vi "Tosca-Init Data Analysis.vi"(0 "Tosca":refnum<class "Parameters.lvclass">, 2 "IPC":T2, 9 "Control Refs":T1, 11 "error in (no error)":errorcluster, 12 "Session Info":T3={"Animal ID"="", "Session"=1, "Path"=path "", "Run"=0} {"Session" min=1 step=1}) -> (3 "Run":i32, 4 "Tosca out":refnum<class "Parameters.lvclass">, 13 "Session Info out":T3={"Animal ID"="", "Session"=1, "Path"=path "", "Run"=0} {"Session" min=1 step=1}, 14 "Analysis":T4, 15 "error out":errorcluster)   [LabVIEW 2020]
uses:
  Typedefs/Tosca-Session Info.ctl
  Typedefs/Tosca-Analysis State.ctl
  Typedefs/Tosca-Adaptation State.ctl
  Typedefs/Tosca-Adaptation Track State.ctl
  Typedefs/Tosca-Adaptation History Element.ctl
  Classes/Parameters/Histogram Data.ctl
  Classes/Parameters/Connect.ctl
  IPC VIs/Tosca-IPC.ctl
  Classes/Parameters/Parameters.lvclass
  Digital Input VIs/Tosca-DI Queue Data.ctl
  Digital Input VIs/Tosca-Input Event.ctl
  Digital Input VIs/Tosca-Input Criterion.ctl
  epl-vi-lib/Utility VIs/Type Defs/Logic State.ctl
  Typedefs/Tosca-Accumulator.ctl
  Typedefs/Tosca-State AODO.ctl
  Typedefs/Tosca-AO Runtime.ctl
  Typedefs/Tosca-DO Runtime.ctl
  epl-vi-lib/Signal Synthesis VIs/4th Generation/Classes/SignalManager/SignalManager.lvclass
  Typedefs/Tosca-Synapse Start Data.ctl
  IPC VIs/Tosca-Message.ctl
  IPC VIs/Tosca-Message Action.ctl
  Typedefs/Tosca-Thread Type.ctl
  Imaging VIs/Tosca-2P-Notifier Data.ctl
  Typedefs/Tosca-MATLAB Queue Data.ctl
  Visual Stim VIs/Tosca-Grating.ctl
  Visual Stim VIs/Tosca-Grating Type.ctl
  Typedefs/Tosca-File IO Notification.ctl
  Typedefs/Tosca-Control Refs.ctl
  FSM Graph VIs/LV Source/FSM Editor/FSM Editor.xctl
  Classes/Parameters/Parameters.lvclass/Parameters.ctl
  Classes/Parameters/Read MATLAB function.vi
  Classes/Parameters/Read Connect.vi
  Classes/Parameters/Read AI.vi
  Tosca-Globals.vi
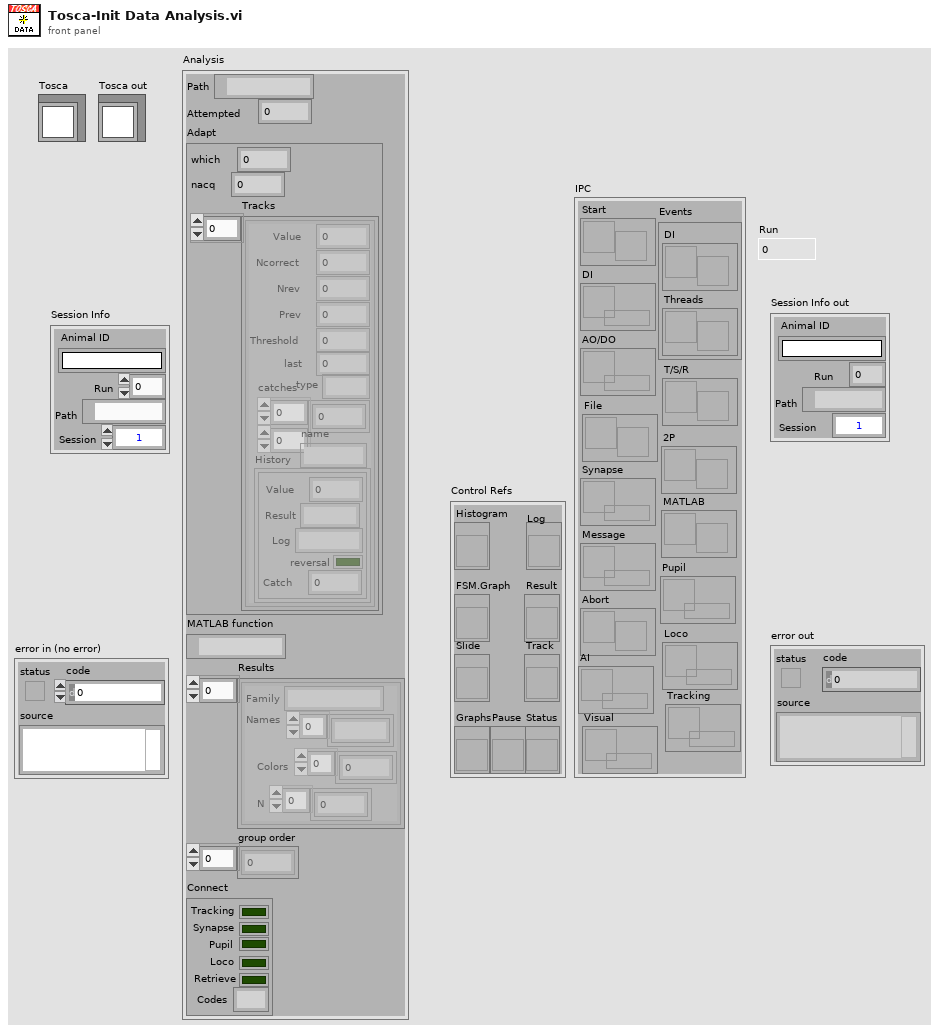
[diagram p1: front panel]
types:
  T1 = typedef "Tosca-Control Refs.ctl" = cluster{"FSM.Graph":refnum<vi>, "Slide":refnum<vi>, "Result":refnum<vi>, "Histogram":refnum<vi>, "Graphs":refnum<vi>, "Track":refnum<vi>, "Log":refnum<vi>, "Status":refnum<vi>, "Pause":refnum<vi>}
  T2 = typedef "Tosca-IPC.ctl" = cluster{"Start":refnum<notifier>, "DI":refnum<queue>, "AO/DO":refnum<queue>, "Synapse":refnum<queue>, "Message":refnum<queue>, "Abort":refnum<notifier>, "Events":cluster{"DI":refnum<user-event>, "Threads ":refnum<user-event>}, "T/S/R":refnum<notifier>, "2P":refnum<notifier>, "MATLAB":refnum<notifier>, "Pupil":refnum<queue>, "Loco":refnum<queue>, "AI":refnum<queue>, "Tracking":refnum<queue>, "Visual":refnum<queue>, "File":refnum<notifier>}
  T3 = typedef "Tosca-Session Info.ctl" = cluster{"Animal ID":string, "Session":i32, "Path":path, "Run":i32}
  T4 = typedef "Tosca-Analysis State.ctl" = cluster{"Path":path, "Attempted":i32, "Adapt":T5, "MATLAB function":path, "Results":T8[], "group order":i32[], "Connect":T9}
  T5 = typedef "Tosca-Adaptation State.ctl" = cluster{"which":i32, "nacq":i32, "Tracks":T6[]}
  T6 = typedef "Tosca-Adaptation Track State.ctl" = cluster{"Value":dbl, "Ncorrect":i32, "Nrev":i32, "Prev":dbl, "History":T7[], "Threshold":dbl, "last":i32, "type":string, "catches":dbl[][], "name":string}
  T7 = typedef "Tosca-Adaptation History Element.ctl" = cluster{"Value":dbl, "Result":string, "Log":string, "reversal":bool, "Catch":dbl}
  T8 = typedef "Parameters.lvclass/Histogram Data.ctl" = cluster{"Family":string, "Names":string[], "Colors":u32[], "N":i32[]}
  T9 = typedef "Parameters.lvclass/Connect.ctl" = cluster{"Tracking":bool, "Synapse":bool, "Pupil":bool, "Loco":bool, "Retrieve":bool, "Codes":string}
  T10 = typedef "Tosca-File IO Notification.ctl" = cluster{"Operation":enum16{"Start", "Update", "Finish"}, "Filestem":string}
  T11 = typedef "Tosca-AI.ctl" = cluster{"active":bool, "Fs":dbl, "AI":string[], "DI":string[]}
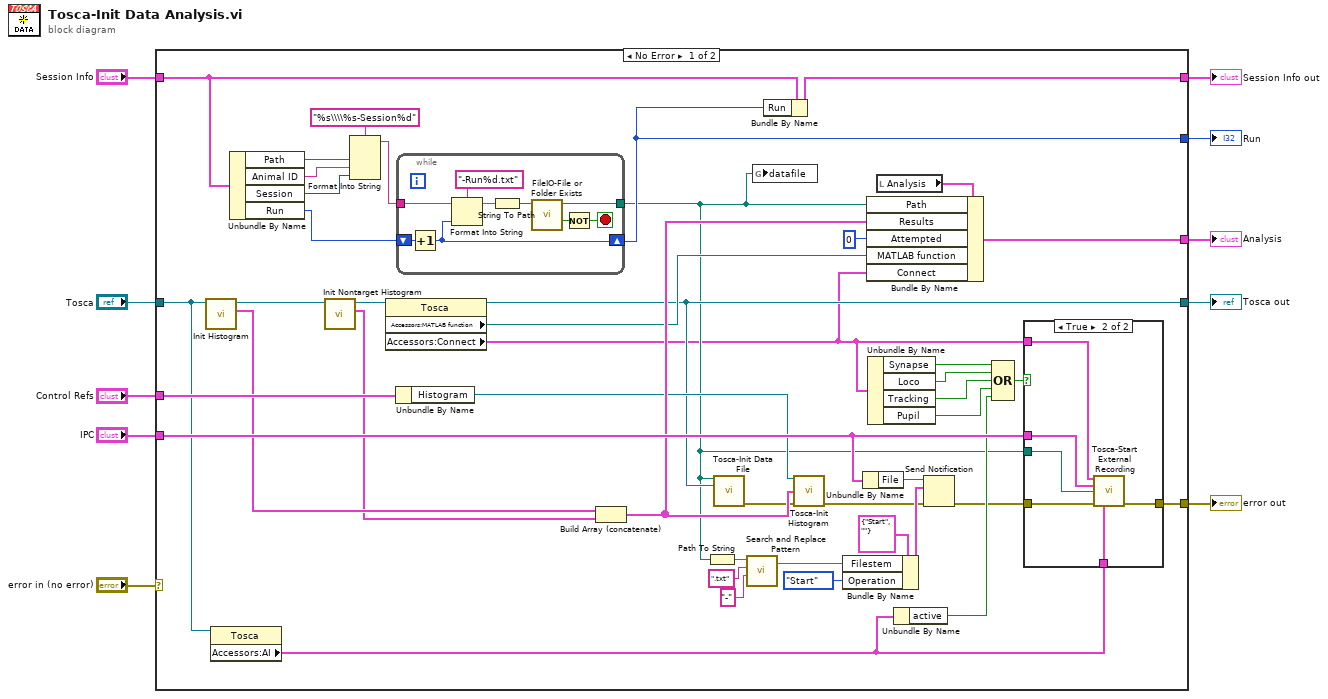
[diagram p0: block diagram]
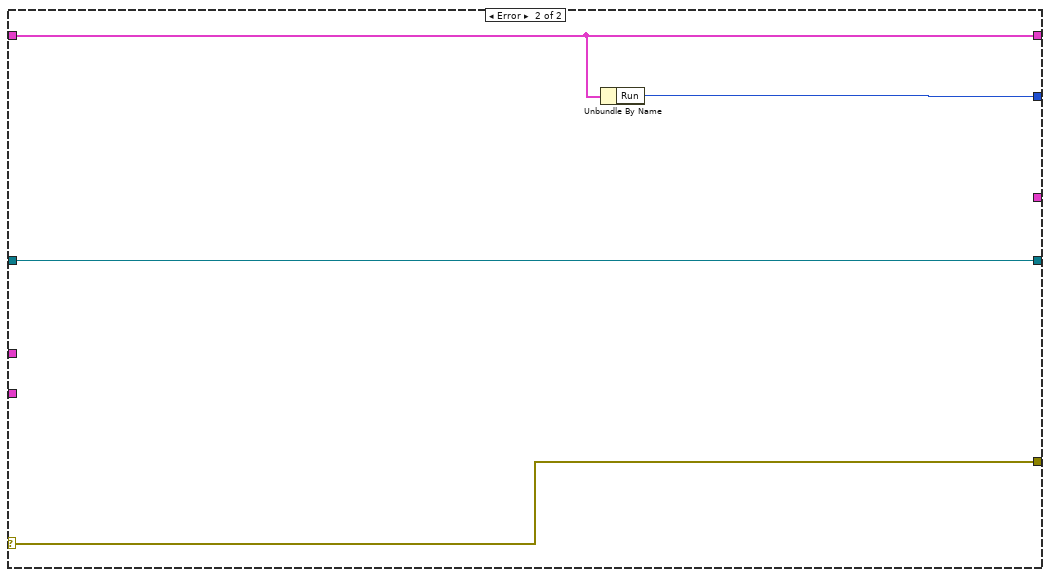
[diagram p3: hidden frame]
diagram:
  n1 = case shown="No Error" "error in (no error)" {
    selector: "error in (no error)" -> [_ w74]
    tunnel: [w34 w74] -> w9
    tunnel: "Session Info" -> [w45 w73]
    tunnel: [w47 _] -> w7
    tunnel: [w44 w73] -> w6
    tunnel: [w37 w72] -> w5
    tunnel: "IPC" -> [w33 _]
    tunnel: "Control Refs" -> [w30 _]
    tunnel: "Tosca" -> [w20 w71]
    tunnel: [w18 w71] -> w1
    frame No Error {
      n2 = call "Init Histogram.vi"("Tosca in"=w20) -> ("Data"=w19:T8[], "Tosca out"=w16:refnum<class "Parameters.lvclass">)  [unwired: 8 in, 1 out]
      n3 = property class="Tosca"(reference=w20) -> ("Accessors:AI"=w21:T11)  [unwired: 1 in, 2 out]
      n4 = Unbundle By Name(w45) -> ("Path"=w53:path, "Animal ID"=w52:string, "Session"=w51:i32, "Run"=w49:i32)
      n5 = call "Init Nontarget Histogram.vi"("Tosca in"=w16) -> ("Data"=w14:T8, "Tosca out"=w15:refnum<class "Parameters.lvclass">)  [unwired: 8 in, 1 out]
      n6 = Format Into String(format string="%s\\\\%s-Session%d", w53, w52, w51) -> (resulting string=w50:string)  [unwired: 2 in, 1 out]
      n7 = property class="Tosca"(reference=w15) -> (reference out=w18:refnum<class "Parameters.lvclass">, "Accessors:MATLAB function"=w23:path, "Accessors:Connect"=w13:T9)  [unwired: 1 in, 1 out]
      n8 = Unbundle By Name(w30) -> ("Histogram"=w29:refnum<vi>)
      n9 = while {
        tunnel: w50 -> [w68]
        tunnel: [w64] -> w17
        shift-right: [w66] -> w37
        shift-left: w49 -> [w67]
        stop <- w63 stop-if-true
        n10 = Increment(x=w67) -> (x+1=w66:i32)
        n11 = Format Into String(format string="-Run%d.txt", initial string=w68, w66) -> (resulting string=w69:string)  [unwired: 1 in, 1 out]
        n12 = String To Path(string=w69) -> (path=w65:path)
        n13 = call "FileIO-File or Folder Exists.vi"("path"=w65) -> ("Exists?"=w62:bool, "dup path"=w64:path)  [unwired: 7 in, 2 out]
        n14 = Not(x=w62) -> (.not. x?=w63:bool)
      }
      n15 = Build Array (concatenate)(w19, w14) -> (w31:T8[])
      n16 = Path To String(path=w17) -> (string=w38:string)
      n17 = call "Tosca-Init Data File.vi"("Path"=w17, "Tosca"=w18) -> ("error out"=w11:errorcluster)  [unwired: 13 in]
      n18 = call <vilib>:"Search and Replace Pattern.vi"("string"=w38, "regular expression (\"\")"=".txt" ("regular expression (\"\")"), "replace string (\"\")"="-" ("replace string (\"\")")) -> ("result string"=w36:string)  [unwired: 2 in, 1 out]
      n19 = global write "Tosca-Globals.vi" "datafile"(w17) -> ()
      n20 = Bundle By Name(cluster=w45, "Run"=w37) -> (w44:T3)
      n21 = call "Tosca-Init Histogram.vi"("Histogram"=w29, "Results"=w31, "error in (no error)"=w11) -> ("error out"=w32:errorcluster)  [unwired: 12 in]
      n22 = Bundle By Name(cluster=T10 {"Operation"=enum."Start", "Filestem"=""} ("element"), "Filestem"=w36, "Operation"=enum16{"Start", "Update", "Finish"}."Start") -> (w42:T10)
      n23 = Unbundle By Name(w33) -> ("File"=w35:refnum<notifier>)
      n24 = Unbundle By Name(w13) -> ("Synapse"=w28:bool, "Loco"=w27:bool, "Tracking"=w25:bool, "Pupil"=w22:bool)
      n25 = local read "Analysis"() -> (w48:T4)
      n26 = Bundle By Name(cluster=w48, "Path"=w17, "Results"=w31, "Attempted"=0, "MATLAB function"=w23, "Connect"=w13) -> (w47:T4)
      n27 = Unbundle By Name(w21) -> ("active"=w24:bool)
      n28 = Send Notification(notification=w42, notifier=w35, error in (no error)=w32) -> (error out=w12:errorcluster)  [unwired: 1 out]
      n29 = Compound Arithmetic op=OR(w28, w27, w25, w22, w24) -> (w26:bool)
      n30 = case shown="True" w26 {
        tunnel: w13 -> [_ w56]
        tunnel: w12 -> [w55 w61]
        tunnel: [w55 w60] -> w34
        tunnel: w33 -> [_ w59]
        tunnel: w17 -> [_ w58]
        tunnel: w21 -> [_ w57]
        frame False {
        }
        frame True {
          n31 = call "Tosca-Start External Recording.vi"("Connect"=w56, "IPC"=w59, "Path"=w58, "error in (no error)"=w61, "AI"=w57) -> ("error out"=w60:errorcluster)  [unwired: 10 in]
        }
      }
    }
    frame Error {
      n32 = Unbundle By Name(w73) -> ("Run"=w72:i32)
    }
  }
  "error out" <- w9
  "Analysis" <- w7
  "Session Info out" <- w6
  "Run" <- w5
  "Tosca out" <- w1
